vi "Build NT RPC Descriptor.vi"(11 "VI in":refnum<vi>) -> (3 "string buffer":string)   [LabVIEW 2017]
uses:
  <vilib>/Utility/Data Type/Type Definitions/Data Type.ctl
  <vilib>/Rock Robotics/Network Tables/Field Type.ctl
  <vilib>/Utility/Data Type/NI_Data Type.lvlib
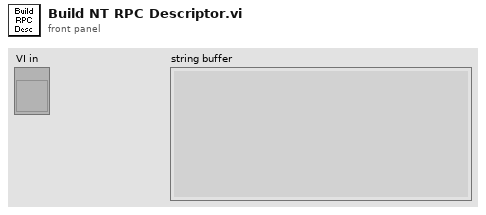
[diagram p1: front panel]
types:
  T1 = typedef "NI_Data Type.lvlib/Data Type.ctl" = enum8{"Invalid Type", "Void", "I8", "I16", "I32", "I64", "U8", "U16", "U32", "U64", "Single Float", "Double Float", "Extended Float", "Single Complex", "Double Complex", "Extended Complex", "Enum U8", "Enum U16", "Enum U32", "Enum U64", "Single Float With Unit", "Double Float With Unit", "Extended Float With Unit", "Single Complex with Unit", "Double Complex with Unit", "Extended Complex with Unit", "Boolean", "String", "Path", "Picture", "Tag", "Array", "Cluster", "Variant", "LV Variant", "Waveform", "Timestamp", "Digital Waveform", "Digital Data", "ExpressData", "Refnum", "External Data", "VI", "Poly VI", "LabVIEW Class Instance", "Fixed Point"}
  T2 = typedef "NI_Data Type.lvlib/VI Info.ctl" = cluster{"Connector Pane Pattern":i16, "Connector Pane Rotation":i16, "Flags":u32[], "Modification Date":timestamp, "Asynchronous":bool, "Non-Function":bool, "Subroutine":bool, "SubSystem":bool}
  T3 = typedef "Field Type.ctl" = enum8{"Invalid", "Bool", "Numeric", "String", "Raw", "Boolean Array", "Numeric Array", "String Array", "RPC"}
  T4 = typedef "NI_Data Type.lvlib/Type Definition Info.ctl" = cluster{"Name":string, "Timestamp":u32}
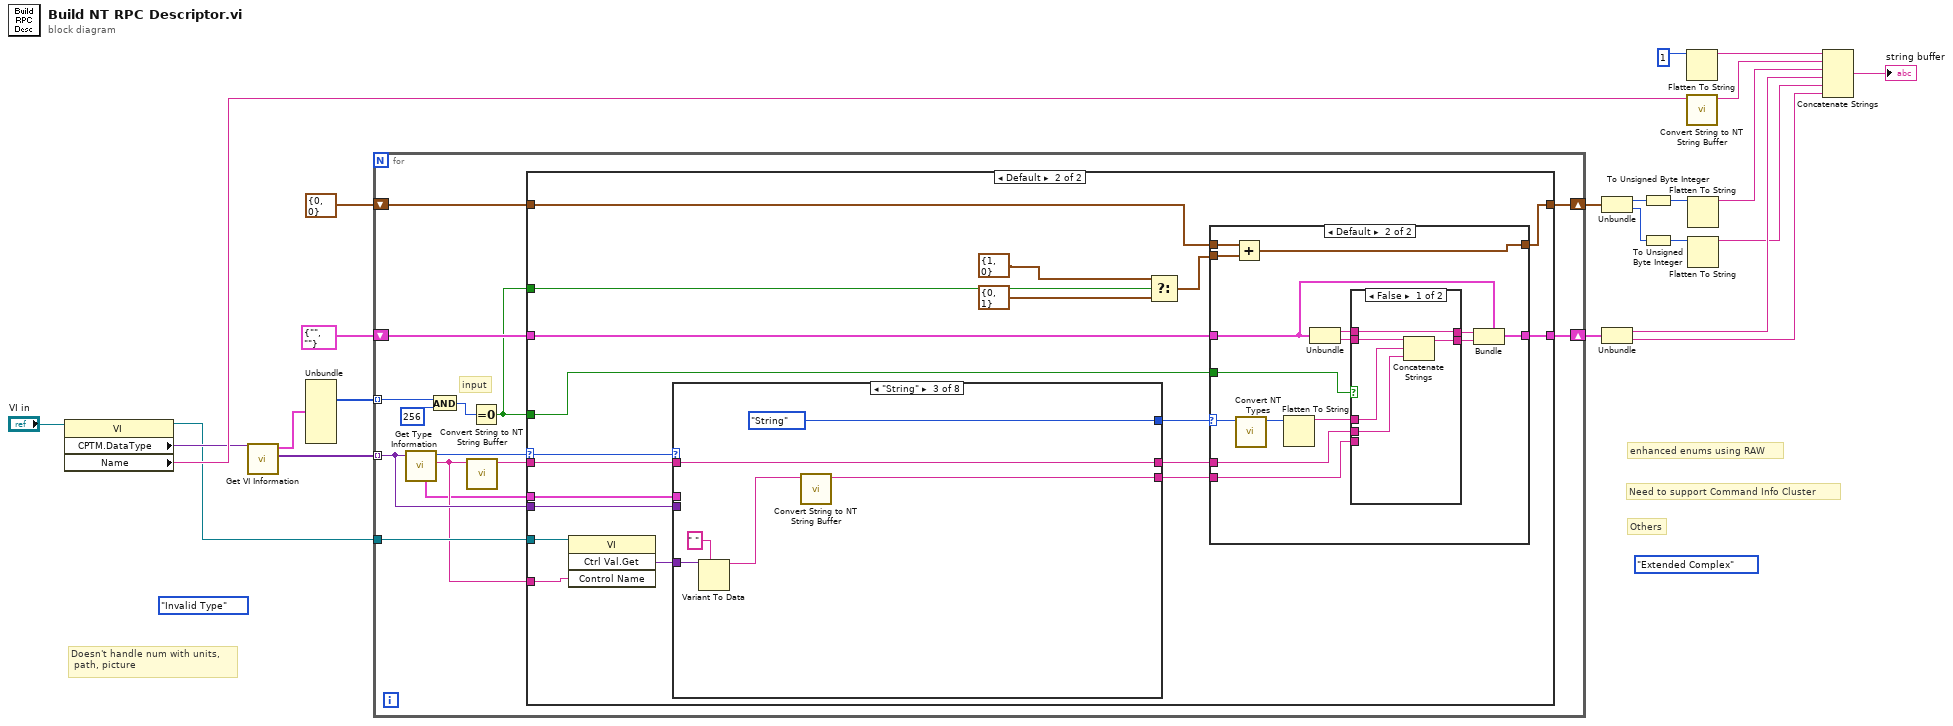
[diagram p0: block diagram]
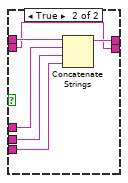
[diagram p4: hidden frame]
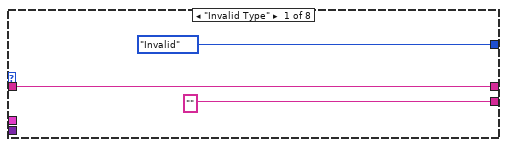
[diagram p5: hidden frame]
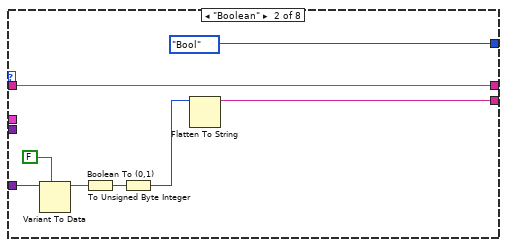
[diagram p6: hidden frame]
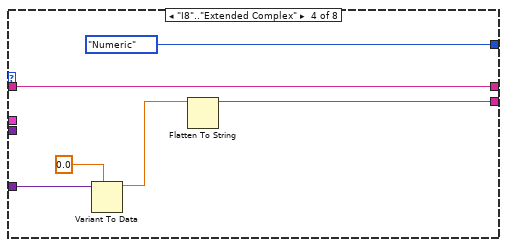
[diagram p7: hidden frame]
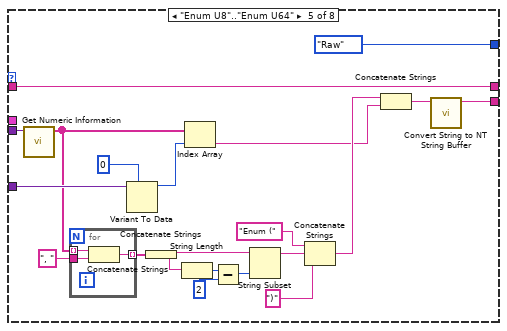
[diagram p8: hidden frame]
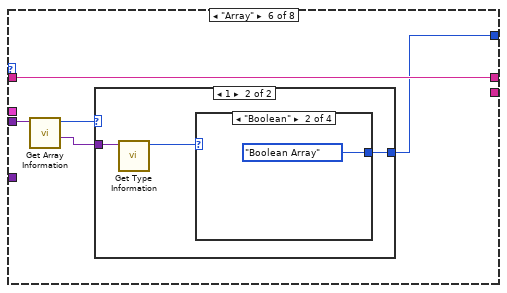
[diagram p9: hidden frame]
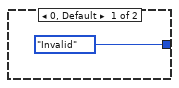
[diagram p10: hidden frame]
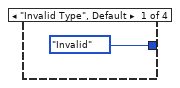
[diagram p11: hidden frame]
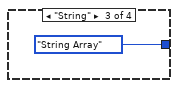
[diagram p12: hidden frame]
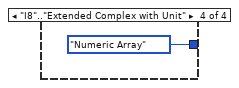
[diagram p13: hidden frame]
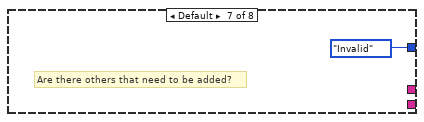
[diagram p14: hidden frame]
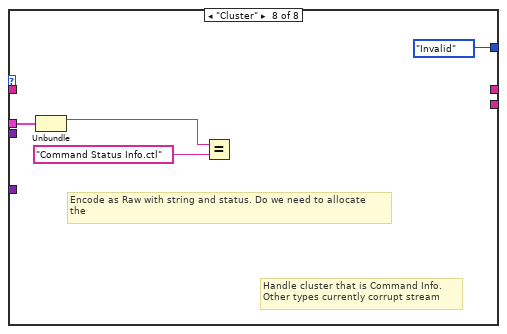
[diagram p15: hidden frame]
diagram:
  (unwired) Data_Type."Invalid Type" ("Type")
  (unwired) Data_Type."Extended Complex" ("Type")
  # "Doesn't handle num with units,\n path, picture"
  # "Need to support Command Info Cluster"
  # "Others"
  # "enhanced enums using RAW"
  n1 = property class="VI"(reference="VI in") -> (reference out=w1:refnum<vi>, "CPTM.DataType"=w16:variant, "Name"=w17:string)  [unwired: 1 in, 1 out]
  n2 = call <vilib>:"Get VI Information.vi"("Variant"=w16) -> ("VI Terminal Types"=w21:variant[], "VI Info"=w14:T2)  [unwired: 7 in, 2 out]
  n3 = Unbundle(w14) -> ("Flags"=w13:u32[])  [unwired: 7 out]
  n4 = for {
    tunnel: w21 -> [w36] mode=indexing
    tunnel: w13 -> [w35] mode=indexing
    shift-right: [w28] -> w10
    shift-left: cluster{u32, u32} {0, 0} -> [w29]
    shift-right: [w30] -> w9
    shift-left: cluster{string, string} {"", ""} -> [w31]
    tunnel: w1 -> [w26]
    # "input"
    n5 = call <vilib>:"Get Type Information.vi"("Variant"=w36) -> ("Name"=w25:string, "Type"=w32:T1, "Type Definition Info"=w24:T4)  [unwired: 6 in, 2 out]
    n6 = And(x=w35, y=u32 256) -> (x .and. y?=w33:u32)
    n7 = call <vilib>:"Convert String to NT String Buffer.vi"("LV Buffer"=w25) -> ("NT Buffer"=w37:string)  [unwired: 10 in]
    n8 = Equal To 0?(x=w33) -> (x = 0?=w27:bool)
    n9 = case shown="Default" w32 {
      selector: w32 -> [_ w57]
      tunnel: w37 -> [_ w49]
      tunnel: w36 -> [_ w58]
      tunnel: w27 -> [_ w56]
      tunnel: w31 -> [w39 w55]
      tunnel: [w39 w54] -> w30
      tunnel: w29 -> [w38 w42]
      tunnel: [w38 w41] -> w28
      tunnel: w27 -> [_ w51]
      tunnel: w26 -> [_ w50]
      tunnel: w25 -> [_ w45]
      tunnel: w24 -> [_ w44]
      frame "Invalid Type", "Void" {
      }
      frame Default {
        n10 = invoke class="VI" method="Ctrl Val.Get"(reference=w50, "Control Name"=w45) -> ("Get Control Value Variant"=w48:variant)  [unwired: 2 in, 3 out]
        n11 = case shown="\"String\"" w57 {
          tunnel: w49 -> [w88 w96 w102 w108 w128 w137 _ _]
          tunnel: [Field_Type."Invalid" ("Type") Field_Type."Bool" ("Type") Field_Type."String" ("Type") Field_Type."Numeric" ("Type") Field_Type."Raw" ("Type") w133 Field_Type."Invalid" ("Type") Field_Type."Invalid" ("Type")] -> w43
          tunnel: [w88 w96 w102 w108 w128 w137 _ _] -> w47
          tunnel: ["" w95 w98 w107 w110 _ _ _] -> w46
          tunnel: w58 -> [_ _ _ _ w125 w136 _ _]
          tunnel: w48 -> [_ w94 w101 w106 w127 _ _ _]
          tunnel: w44 -> [_ _ _ _ _ _ _ w149]
          frame "Invalid Type" {
          }
          frame "Boolean" {
            n12 = Variant To Data(type=FALSE, Variant=w94) -> (data=w92:bool)  [unwired: 1 in, 1 out]
            n13 = Boolean To (0,1)(Boolean=w92) -> (0, 1=w91:i16)
            n14 = To Unsigned Byte Integer(number=w91) -> (unsigned 8bit integer=w90:u8)
            n15 = Flatten To String(anything=w90) -> (data string=w95:string)  [unwired: 3 in, 2 out]
          }
          frame "String" {
            n16 = Variant To Data(type=" ", Variant=w101) -> (data=w99:string)  [unwired: 1 in, 1 out]
            n17 = call <vilib>:"Convert String to NT String Buffer.vi"("LV Buffer"=w99) -> ("NT Buffer"=w98:string)  [unwired: 10 in]
          }
          frame "I8".."Extended Complex" {
            n18 = Variant To Data(type=0.0, Variant=w106) -> (data=w104:dbl)  [unwired: 1 in, 1 out]
            n19 = Flatten To String(anything=w104) -> (data string=w107:string)  [unwired: 3 in, 2 out]
          }
          frame "Enum U8".."Enum U64" {
            n20 = call <vilib>:"Get Numeric Information.vi"("Variant"=w125) -> ("Enum Names"=w112:string[])  [unwired: 7 in, 3 out]
            n21 = for {
              tunnel: w112 -> [w132] mode=indexing
              tunnel: [w131] -> w122 mode=indexing
              tunnel: ", " ("format string") -> [w130]
              n22 = Concatenate Strings(w132, w130) -> (w131:string)
            }
            n23 = Variant To Data(type=u32 0, Variant=w127) -> (data=w124:u32)  [unwired: 1 in, 1 out]
            n24 = Concatenate Strings(w122) -> (w123:string)
            n25 = String Length(string=w123) -> (length=w120:i32)
            n26 = Index Array(array=w112, index=w124) -> (element=w113:string)
            n27 = Subtract(x=w120, y=u32 2) -> (x-y=w119:u32)
            n28 = String Subset(string=w123, length (rest)=w119) -> (substring=w117:string)  [unwired: 1 in]
            n29 = Concatenate Strings("Enum (" ("format string"), w117, ")" ("format string")) -> (w114:string)
            n30 = Concatenate Strings(w114, w113) -> (w111:string)
            n31 = call <vilib>:"Convert String to NT String Buffer.vi"("LV Buffer"=w111) -> ("NT Buffer"=w110:string)  [unwired: 10 in]
          }
          frame "Array" {
            n32 = call <vilib>:"Get Array Information.vi"("Variant"=w136) -> ("Array Element Data Type"=w134:variant, "Number of Dimensions"=w135:i32)  [unwired: 7 in, 2 out]
            n33 = case shown="1" w135 {
              tunnel: w134 -> [_ w141]
              tunnel: [Field_Type."Invalid" ("Type") w139] -> w133
              frame 0, Default {
              }
              frame 1 {
                n34 = call <vilib>:"Get Type Information.vi"("Variant"=w141) -> ("Type"=w140:T1)  [unwired: 6 in, 4 out]
                n35 = case shown="\"Boolean\"" w140 {
                  tunnel: [Field_Type."Invalid" ("Type") Field_Type."Boolean Array" ("Type") Field_Type."String Array" ("Type") Field_Type."Numeric Array" ("Type")] -> w139
                  frame "Invalid Type", Default {
                  }
                  frame "Boolean" {
                  }
                  frame "String" {
                  }
                  frame "I8".."Extended Complex with Unit" {
                  }
                }
              }
            }
          }
          frame Default {
            # "Are there others that need to be added?"
          }
          frame "Cluster" {
            # "Encode as Raw with string and status. Do we need to allocate\nthe"
            # "Handle cluster that is Command Info.\nOther types currently corrupt stream"
            n36 = Unbundle(w149) -> ("Name"=w147:string)  [unwired: 1 out]
            n37 = Equal?(x=w147, y="Command Status Info.ctl" ("Name")) -> ()  [unwired: 1 out]
          }
        }
        n38 = Select(t=cluster{u32, u32} {1, 0}, s=w51, f=cluster{u32, u32} {0, 1}) -> (s? t:f=w40:cluster{u32, u32})
        n39 = case shown="Default" w43 {
          selector: w43 -> [_ w64]
          tunnel: w56 -> [_ w74]
          tunnel: w55 -> [w60 w73]
          tunnel: [w60 w72] -> w54
          tunnel: w47 -> [_ w66]
          tunnel: w46 -> [_ w65]
          tunnel: w42 -> [w59 w63]
          tunnel: [w59 w61] -> w41
          tunnel: w40 -> [_ w62]
          frame "Invalid" {
          }
          frame Default {
            n40 = Add(x=w63, y=w62) -> (x+y=w61:cluster{u32, u32})
            n41 = call <vilib>:"Convert NT Types.vi"("Type in"=w64) -> ("Type out"=w75:u8)  [unwired: 10 in]
            n42 = Flatten To String(anything=w75) -> (data string=w67:string)  [unwired: 3 in, 2 out]
            n43 = Unbundle(w73) -> (w71:string, w70:string)
            n44 = case shown="False" w74 {
              tunnel: w67 -> [w77 w84]
              tunnel: w71 -> [w78 w86]
              tunnel: w70 -> [w80 w83]
              tunnel: [w78 w85] -> w69
              tunnel: [w79 w83] -> w68
              tunnel: w66 -> [w76 w82]
              tunnel: w65 -> [_ w81]
              frame False {
                n45 = Concatenate Strings(w80, w77, w76) -> (w79:string)
              }
              frame True {
                n46 = Concatenate Strings(w86, w84, w82, w81) -> (w85:string)
              }
            }
            n47 = Bundle(cluster=w73, w69, w68) -> (w72:cluster{string, string})
          }
        }
      }
    }
  }
  n48 = Unbundle(w10) -> (w8:u32, w6:u32)
  n49 = Unbundle(w9) -> (w4:string, w2:string)
  n50 = To Unsigned Byte Integer(number=w8) -> (unsigned 8bit integer=w22:u8)
  n51 = To Unsigned Byte Integer(number=w6) -> (unsigned 8bit integer=w7:u8)
  n52 = Flatten To String(anything=u8 1) -> (data string=w19:string)  [unwired: 3 in, 2 out]
  n53 = call <vilib>:"Convert String to NT String Buffer.vi"("LV Buffer"=w17) -> ("NT Buffer"=w20:string)  [unwired: 10 in]
  n54 = Flatten To String(anything=w22) -> (data string=w23:string)  [unwired: 3 in, 2 out]
  n55 = Flatten To String(anything=w7) -> (data string=w3:string)  [unwired: 3 in, 2 out]
  n56 = Concatenate Strings(w19, w20, w23, w4, w3, w2) -> (→"string buffer":string)
